vi "Write Log Instance.vi"(10 "oggerReference.":refnum<class "LoggerReference.lvclass">, 11 "Logger in":refnum<class "Logger.lvclass">) -> (3 "Logger out":refnum<class "Logger.lvclass">)   [LabVIEW 2020, in "Event Log.lvlib" / "Logger.lvclass"]
uses:
  Logger.lvclass
  <vilib>/gpm_packages/@cs/event-logger/Source/Composed Log/LoggerReference/LoggerReference.lvclass
  Logger.lvclass/Logger.ctl
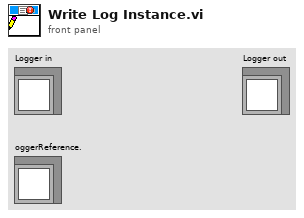
[diagram p1: front panel]
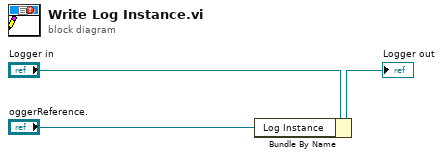
[diagram p0: block diagram]
diagram:
  n1 = Bundle By Name(cluster="Logger in", "Log Instance"="oggerReference.") -> (→"Logger out":refnum<class "Logger.lvclass">)
